vi "Set Full Image.vi"(10 "vbin":i32, 11 "hbin":i32) -> (3 "function return":u32)   [LabVIEW 2018, in "Copy of Andor SDK.lvlib"]
doc: "EXPNETTYPE unsigned int WINAPI SetFullImage(int hbin, int vbin);"
uses:
  Copy of Andor SDK.lvlib
  <userlib>/Andor SDK/ATMCD32D.dll
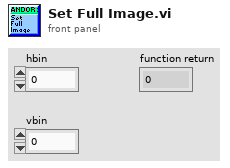
[diagram p1: front panel]
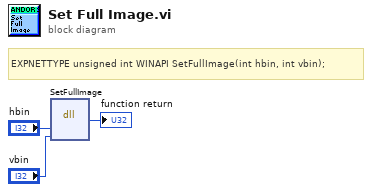
[diagram p0: block diagram]
diagram:
  # "EXPNETTYPE unsigned int WINAPI SetFullImage(int hbin, int vbin);"
  n1 = dll-call lib="C:/Program Files (x86)/National Instruments/LabVIEW 2018/user.lib/Andor SDK/ATMCD32D.*" fn="SetFullImage"("hbin"="hbin", "vbin"="vbin") -> (→"function return":u32)  [unwired: 5 in, 2 out]
